vi "Configure Timebase.vi"(7 "Record Length (10: 10k points)":u32(ring)=10 items=["1000 points"=1, "10k points"=10, "100k points"=100, "1M points"=1000, "5M points"=5000, "10M points"=10000], 8 "error in (no error)":errorcluster, 9 "Position (10 %)":dbl=10.0, 10 "Timebase (0.0005 s)":dbl=0.0005, 11 "VISA resource name":refnum<visa-resource-name>) -> (0 "error out":errorcluster, 3 "VISA resource name out":refnum<visa-resource-name>)   [LabVIEW 2013, in "Tektronix DPO MSO 2000 4000 Series.lvlib"]
doc: "Configures the timebase and horizontal properties of the oscilloscope."
uses:
  Tektronix DPO MSO 2000 4000 Series.lvlib
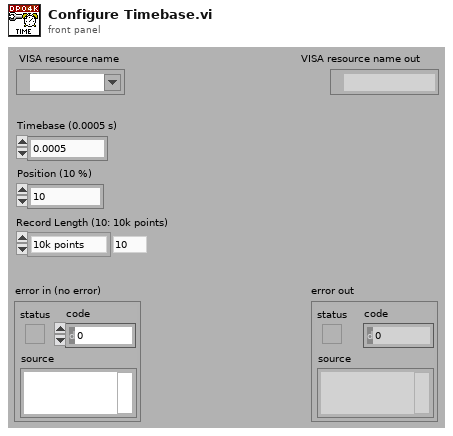
[diagram p1: front panel]
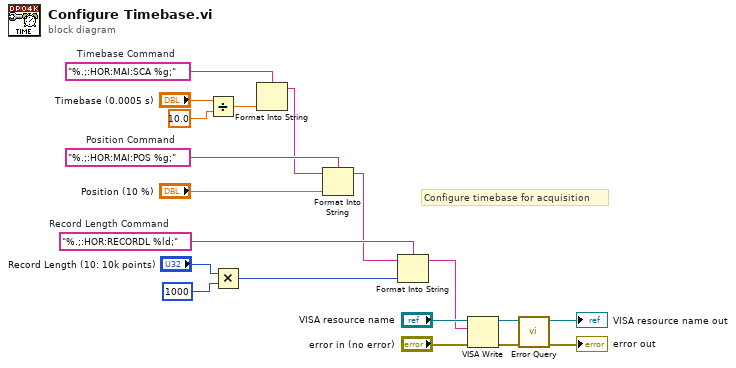
[diagram p0: block diagram]
diagram:
  w9 = "%.;:HOR:RECORDL %ld;"  # Record Length Command
  w12 = "%.;:HOR:MAI:POS %g;"  # Position Command
  w13 = "%.;:HOR:MAI:SCA %g;"  # Timebase Command
  # "Configure timebase for acquisition"
  n1 = Divide(x="Timebase (0.0005 s)", y=10.0) -> (x/y=w2:dbl)
  n2 = Multiply(x="Record Length (10: 10k points)", y=u16 1000) -> (x*y=w6:u32)
  n3 = Format Into String(format string=w13, w2) -> (resulting string=w11:string)  [unwired: 2 in, 1 out]
  n4 = Format Into String(format string=w12, initial string=w11, "Position (10 %)") -> (resulting string=w8:string)  [unwired: 1 in, 1 out]
  n5 = Format Into String(format string=w9, initial string=w8, w6) -> (resulting string=w5:string)  [unwired: 1 in, 1 out]
  n6 = VISA Write(VISA resource name="VISA resource name", write buffer=w5, error in (no error)="error in (no error)") -> (VISA resource name out=w15:refnum<visa-resource-name>, error out=w14:errorcluster)  [unwired: 1 out]
  n7 = call "Error Query.vi"("error in (no error)"=w14, "VISA resource name"=w15) -> ("error out"=→"error out":errorcluster, "VISA resource name out"=→"VISA resource name out":refnum<visa-resource-name>)  [unwired: 6 in, 2 out]
